vi "start.vi"(8 "error in (no error)":errorcluster, 11 "ClockDL100201DAQmx in":refnum<class "ClockMT120808DAQmxSimple.lvclass">) -> (0 "error out":errorcluster, 3 "ClockDL100201DAQmx out":refnum<class "ClockMT120808DAQmxSimple.lvclass">)   [LabVIEW 2010, in "ClockMT120808DAQmxSimple.lvclass"]
doc: "Starts the generation of the pulse trains or, if configured, arms the trigger for the operation to start"
uses:
  ClockMT120808DAQmxSimple.lvclass
  GenericClock/GenericClock/GenericClock.lvclass
  ClockMT120808DAQmxSimple.lvclass/ClockMT120808DAQmxSimple.ctl
  <vilib>/DAQmx/create/channels.llb/DAQmx Create Channel (CO-Pulse Generation-Frequency).vi
  <vilib>/DAQmx/configure/trigger.llb/DAQmx Start Trigger (None).vi
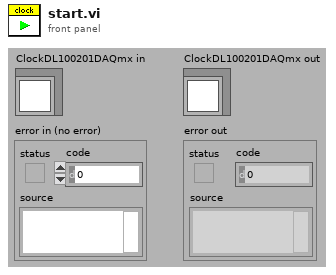
[diagram p1: front panel]
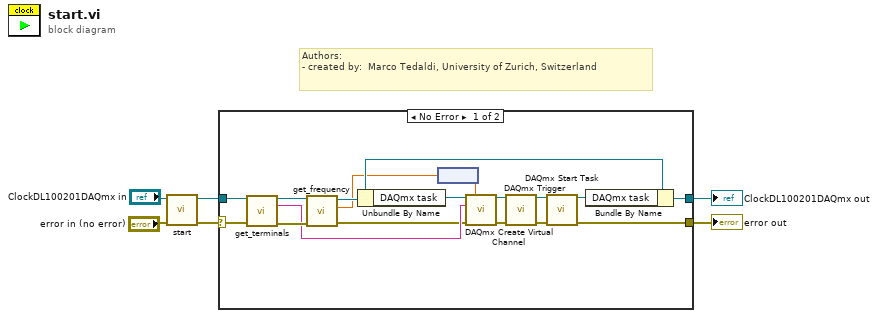
[diagram p0: block diagram]
diagram:
  # "Authors: \n- created by:  Marco Tedaldi, University of Zurich, Switzerland"
  n1 = call-parent "start.vi"("error in (no error)"="error in (no error)", "GenericClock in"="ClockDL100201DAQmx in") -> ("error out"=w4:errorcluster, "GenericClock out"=w3:refnum<class "ClockMT120808DAQmxSimple.lvclass">)  [unwired: 8 in]
  n2 = case shown="No Error" w4 {
    selector: w4 -> [w19 w24]
    tunnel: w3 -> [w20 w25]
    tunnel: [w23 w25] -> w2
    tunnel: [w21 w24] -> w1
    frame No Error {
      n3 = call "get_terminals.vi"("ClockDL100201DAQmx in"=w20, "error in (no error)"=w19) -> ("ClockDL100201DAQmx out"=w18:refnum<class "ClockMT120808DAQmxSimple.lvclass">, "counter"=w11:tag, "error out"=w16:errorcluster)  [unwired: 11 in]
      n4 = call-dynamic "get_frequency.vi"("error in (no error)"=w16, "GenericClock.lvclass in"=w18) -> ("error out"=w10:errorcluster, "frequency"=w15:dbl[unit], "GenericClock.lvclass out"=w17:refnum<class "ClockMT120808DAQmxSimple.lvclass">)  [unwired: 7 in]
      n5 = Unbundle By Name(w17) -> ("DAQmx task"=w12:refnum<k21>)
      n6 = node(w15) -> (w8:dbl)
      n7 = call-poly <vilib>:"DAQmx Create Virtual Channel.vi"("task in"=w12, "frequency"=w8, "counter"=w11, "error in"=w10) -> ("task out"=w7:refnum<k21>, "error out"=w9:errorcluster)  [unwired: 10 in]
      n8 = call-poly <vilib>:"DAQmx Trigger.vi"("task/channels in"=w7, "error in"=w9) -> ("task out"=w14:refnum<k21>, "error out"=w13:errorcluster)  [unwired: 12 in]
      n9 = call <vilib>:"DAQmx Start Task.vi"("task/channels in"=w14, "error in"=w13) -> ("task out"=w22:refnum<k21>, "error out"=w21:errorcluster)  [unwired: 12 in]
      n10 = Bundle By Name(cluster=w17, "DAQmx task"=w22) -> (w23:refnum<class "ClockMT120808DAQmxSimple.lvclass">)
    }
    frame Error {
    }
  }
  "error out" <- w1
  "ClockDL100201DAQmx out" <- w2
